vi "SCTL Sector Accumulation.vi"() -> (3 "New Data?":bool)   [LabVIEW 2013]
uses:
  <vilib>/rvi/FIFO/Fifo_Resource/nirvififoEmulationReadFpgaImpl.vi
  <vilib>/rvi/DataTransferAndStorage/Container/Common/niFpgaContainerGetUniqueNameForEmu.vi
  <vilib>/rvi/Memory/Memory_Emulation/nirvimemoryFastEmulationFpgaImpl.vi
  <instcachedir>/0/nirvimemoryFastEmulationFpgaImpl_5FBAB50466BC4C939F684F8805638BFC.lvgen/nirvimemoryFastEmulationFpgaImpl_5FBAB50466BC4C939F684F8805638BFC_011.vi
  <vilib>/rvi/Memory/Memory_Emulation/nirvimemoryFastEmulation.vi
  <vilib>/rvi/Memory/Memory_Emulation/nirvimemoryEmulation.vi
  <vilib>/rvi/DataTransferAndStorage/Container/XNode/niFpgaContainer.xnode
  <vilib>/rvi/FIFO/Fifo_Resource/nirvififoEmulationRead.vi
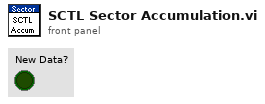
[diagram p1: front panel]
types:
  T1 = cluster{"Accumulated Intensity":u32, "Count":u16}
  T2 = cluster{"Accumulated Intensity":u32, "Count":u16}[]
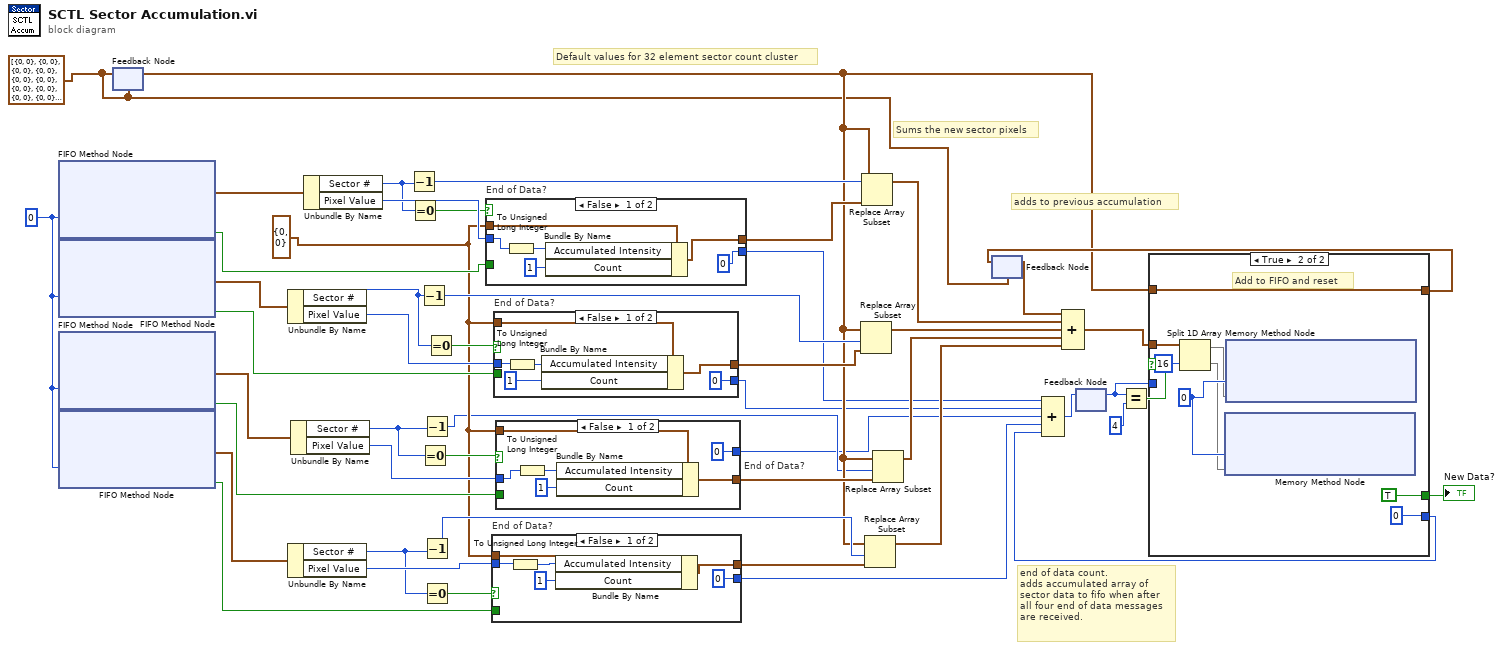
[diagram p0: block diagram]
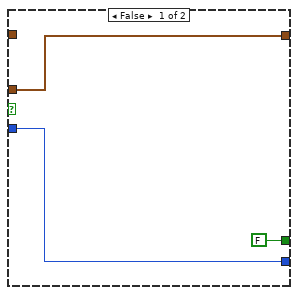
[diagram p2: hidden frame]
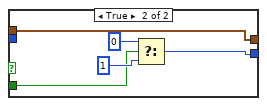
[diagram p3: hidden frame]
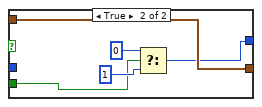
[diagram p4: hidden frame]
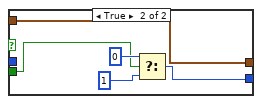
[diagram p5: hidden frame]
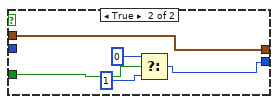
[diagram p6: hidden frame]
diagram:
  w17 = T1 {"Accumulated Intensity"=0, "Count"=0} ("Accumulated Sector Cluster")
  w14 = T2 [{"Accumulated Intensity"=0, "Count"=0}, {"Accumulated Intensity"=0, "Count"=0}, {"Accumulated Intensity"=0, "Count"=0}, {"Accumulated Intensity"=0, "Count"=0}, {"Accumulated Intensity"=0, "Count"=0}, {"Accumulated Intensity"=0, "Count"=0}, {"Accumulated Intensity"=0, "Count"=0}, {"Accumulated Intensity"=0, "Count"=0}, {"Accumulated Intensity"=0, "Count"=0}, {"Accumulated Intensity"=0, "Count"=0}, {"Accumulated Intensity"=0, "Count"=0}, {"Accumulated Intensity"=0, "Count"=0}, {"Accumulated Intensity"=0, "Count"=0}, {"Accumulated Intensity"=0, "Count"=0}, {"Accumulated Intensity"=0, "Count"=0}, {"Accumulated Intensity"=0, "Count"=0}, {"Accumulated Intensity"=0, "Count"=0}, {"Accumulated Intensity"=0, "Count"=0}, {"Accumulated Intensity"=0, "Count"=0}, {"Accumulated Intensity"=0, "Count"=0}, {"Accumulated Intensity"=0, "Count"=0}, {"Accumulated Intensity"=0, "Count"=0}, {"Accumulated Intensity"=0, "Count"=0}, {"Accumulated Intensity"=0, "Count"=0}, {"Accumulated Intensity"=0, "Count"=0}, {"Accumulated Intensity"=0, "Count"=0}, {"Accumulated Intensity"=0, "Count"=0}, {"Accumulated Intensity"=0, "Count"=0}, {"Accumulated Intensity"=0, "Count"=0}, {"Accumulated Intensity"=0, "Count"=0}, {"Accumulated Intensity"=0, "Count"=0}, {"Accumulated Intensity"=0, "Count"=0}] ("Data")
  w49 = 0 ("Timeout")
  # "end of data count.\nadds accumulated array of\nsector data to fifo when after\nall four end of data messages\nare received."
  # "adds to previous accumulation"
  # "Sums the new sector pixels"
  # "Default values for 32 element sector count cluster"
  n1 = xnode ("FIFO Method Node")("Timeout"=w49) -> ("Element"=w48:cluster{"Sector #":u8, "Pixel Value":u8}, "Timed Out?"=w21:bool)  [unwired: 1 in, 1 out]
  n2 = xnode ("FIFO Method Node")("Timeout"=w49) -> ("Element"=w47:cluster{"Sector #":u8, "Pixel Value":u8}, "Timed Out?"=w20:bool)  [unwired: 1 in, 1 out]
  n3 = xnode ("FIFO Method Node")("Timeout"=w49) -> ("Element"=w46:cluster{"Sector #":u8, "Pixel Value":u8}, "Timed Out?"=w19:bool)  [unwired: 1 in, 1 out]
  n4 = xnode ("FIFO Method Node")("Timeout"=w49) -> ("Element"=w45:cluster{"Sector #":u8, "Pixel Value":u8}, "Timed Out?"=w18:bool)  [unwired: 1 in, 1 out]
  n5 = feedback #1(w14) -> (w16:T2)
  n6 = feedback-in #1(w14) -> ()
  n7 = Unbundle By Name(w47) -> ("Sector #"=w31:u8, "Pixel Value"=w41:u8)
  n8 = Unbundle By Name(w45) -> ("Sector #"=w27:u8, "Pixel Value"=w35:u8)
  n9 = Unbundle By Name(w46) -> ("Sector #"=w29:u8, "Pixel Value"=w38:u8)
  n10 = Unbundle By Name(w48) -> ("Sector #"=w33:u8, "Pixel Value"=w43:u8)
  n11 = Decrement(x=w33) -> (x-1=w44:u8)
  n12 = Equal To 0?(x=w33) -> (x = 0?=w32:bool)
  n13 = Decrement(x=w31) -> (x-1=w40:u8)
  n14 = Equal To 0?(x=w29) -> (x = 0?=w28:bool)
  n15 = Decrement(x=w29) -> (x-1=w13:u8)
  n16 = Decrement(x=w27) -> (x-1=w37:u8)
  n17 = Equal To 0?(x=w27) -> (x = 0?=w26:bool)
  n18 = Equal To 0?(x=w31) -> (x = 0?=w30:bool)
  n19 = case "End of Data?" shown="False" w32 {
    tunnel: w43 -> [w51 _]
    tunnel: [w55 w60] -> w42
    tunnel: w17 -> [w54 w60]
    tunnel: [u8 0 w56] -> w5
    tunnel: w21 -> [_ w59]
    frame False {
      n20 = To Unsigned Long Integer(number=w51) -> (unsigned 32bit integer=w50:u32)
      n21 = Bundle By Name(cluster=w54, "Accumulated Intensity"=w50, "Count"=u16 1) -> (w55:T1)
    }
    frame True {
      n22 = Select(t=u8 0, s=w59, f=u8 1) -> (s? t:f=w56:u8)
    }
  }
  n23 = case "End of Data?" shown="False" w26 {
    tunnel: [w66 w71] -> w36
    tunnel: w17 -> [w65 w71]
    tunnel: w35 -> [w62 _]
    tunnel: [u8 0 w67] -> w2
    tunnel: w18 -> [_ w68]
    frame False {
      n24 = To Unsigned Long Integer(number=w62) -> (unsigned 32bit integer=w61:u32)
      n25 = Bundle By Name(cluster=w65, "Accumulated Intensity"=w61, "Count"=u16 1) -> (w66:T1)
    }
    frame True {
      n26 = Select(t=u8 0, s=w68, f=u8 1) -> (s? t:f=w67:u8)
    }
  }
  n27 = case "End of Data?" shown="False" w30 {
    tunnel: w41 -> [w73 _]
    tunnel: w17 -> [w77 w82]
    tunnel: [w76 w82] -> w34
    tunnel: [u8 0 w78] -> w4
    tunnel: w20 -> [_ w79]
    frame False {
      n28 = To Unsigned Long Integer(number=w73) -> (unsigned 32bit integer=w72:u32)
      n29 = Bundle By Name(cluster=w77, "Accumulated Intensity"=w72, "Count"=u16 1) -> (w76:T1)
    }
    frame True {
      n30 = Select(t=u8 0, s=w79, f=u8 1) -> (s? t:f=w78:u8)
    }
  }
  n31 = case "End of Data?" shown="False" w28 {
    tunnel: [w88 w93] -> w39
    tunnel: w38 -> [w84 _]
    tunnel: w17 -> [w87 w93]
    tunnel: [u8 0 w89] -> w3
    tunnel: w19 -> [_ w90]
    frame False {
      n32 = To Unsigned Long Integer(number=w84) -> (unsigned 32bit integer=w83:u32)
      n33 = Bundle By Name(cluster=w87, "Accumulated Intensity"=w83, "Count"=u16 1) -> (w88:T1)
    }
    frame True {
      n34 = Select(t=u8 0, s=w90, f=u8 1) -> (s? t:f=w89:u8)
    }
  }
  n35 = Replace Array Subset(array=w16, new element=w34, index=w40) -> (w9:T2)
  n36 = Replace Array Subset(array=w16, new element=w42, index=w44) -> (w10:T2)
  n37 = Replace Array Subset(array=w16, new element=w36, index=w37) -> (w7:T2)
  n38 = Replace Array Subset(array=w16, new element=w39, index=w13) -> (w8:T2)
  n39 = feedback #2(w14) -> (w12:T2)
  n40 = Compound Arithmetic op=ADD(w12, w10, w9, w8, w7) -> (w11:T2)
  n41 = feedback #3() -> (w23:u8)  [unwired: 1 in]
  n42 = Equal?(x=w23, y=u8 4) -> (x = y?=w24:bool)
  n43 = case shown="True" w24 {
    tunnel: w11 -> [w95 w101]
    tunnel: [w96 u8 0] -> w1
    tunnel: w23 -> [w96 _]
    tunnel: [w95 w103] -> w22
    tunnel: w16 -> [_ w103]
    tunnel: [FALSE ("New Data?") TRUE ("New Data?")] -> w15
    frame False {
    }
    frame True {
      w102 = 0 ("Timeout")
      # "Add to FIFO and reset"
      n44 = Split 1D Array(array=w101, index=16) -> (first subarray=w99:T2, second subarray=w98:T2)
      n45 = xnode ("Memory Method Node")("Address"=w102, "Data"=w98) -> ()  [unwired: 1 in, 1 out]
      n46 = xnode ("Memory Method Node")("Address"=w102, "Data"=w99) -> ()  [unwired: 1 in, 1 out]
    }
  }
  "New Data?" <- w15
  n47 = feedback-in #2(w22) -> ()
  n48 = Compound Arithmetic op=ADD(w5, w4, w3, w2, w1) -> (w6:u8)
  n49 = feedback-in #3(w6) -> ()
